vi "Instrument - Tool.vi"() -> ()   [LabVIEW 2019, in "Instrument Workspace Tool.lvlib"]
uses:
  Instrument Workspace Tool.lvlib
  NationalInstruments.VeriStand.SystemStorage
  Shared/Types/Response Wait Type.ctl
  Workspace Shared/Types/State Variables.ctl
  <vilib>/NI VeriStand/Display Template Support/DisplayTemplateSupport.llb/enum_Display Template Handler Minimal To Workspace.ctl
  <vilib>/NI VeriStand/Display Template Support/DisplayTemplateSupport.llb/enum_Display Template Handler Minimal To Widget Msg.ctl
  <vilib>/NI VeriStand/Execution/Workspace/WorkspaceAPI.ctl
  <vilib>/NI/STM/TCP/TCP Connection Info.ctl
  <vilib>/NI/STM/SubVIs/MetaDataElement.ctl
  Workspace Shared/Types/CD Saved State.ctl
  <vilib>/NI VeriStand/Execution/Workspace/SystemStateEventRef.ctl
  <vilib>/NI VeriStand/Execution/Workspace/Target State Info.ctl
  <vilib>/NI VeriStand/Execution/Workspace/Target State.ctl
  <vilib>/NI VeriStand/Execution/Workspace/SystemStateRegEventRef.ctl
  Shared/Types/Buffered RT Instrument Command.ctl
  <vilib>/NI VeriStand/Execution/Workspace/NI_VS Workspace ExecutionAPI.lvlib
  Host API/Instrument CD Host API.lvlib
  Shared/Instrument Addon Shared.lvlib
  <vilib>/NI/STM/NI STM.lvlib
  Workspace Shared/Instrument Workspace Shared.lvlib
  NationalInstruments.VeriStand.ClientAPI
panel:
  in  "Command":string
  in  "Response?":bool
  in  "Wait Type":T1
  in  "Wait Value":dbl=100.0 format="%#_p"
  out "Timed Out?":bool
  out "Error Report":errorcluster
  out "Response":string
  in  "Send":bool
  out "Device":string
  in  "NIVS.Gateway IP Address":string
  in  "NIVS.System Definition Root":refnum<k24>
  in  "NIVS.Workspace Event":refnum<event-registration>
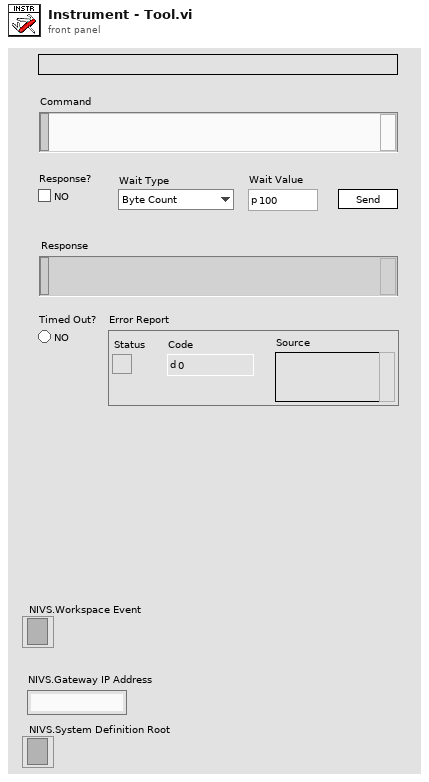
[diagram p1: front panel]
types:
  T1 = typedef "Instrument Addon Shared.lvlib/Response Wait Type.ctl" = enum16{"Byte Count", "Wait sec"}
  T2 = typedef "Instrument Workspace Shared.lvlib/State Variables.ctl" = cluster{"UI.Device":refnum<vi>, "NIVS.CachedDataRef":refnum<user-event>, "NIVS.LaunchRef":refnum<user-event>, "NIVS.SysDefRoot":refnum<k24>, "NIVS.Workspace":T3, "connection info":T4, "NIVS.CachedData":T6, "NIVS.SystemStateRefs":T7, "NIVS.UserEventRefs":cluster{"WorkspaceEvent":refnum<event-registration>, "SystemChangeEventRef":T8, "LaunchRef":refnum<event-registration>}, "Workspace.Connected?":bool, "NIVS.Workspace Event":refnum<event-registration>}
  T3 = typedef "NI_VS Workspace ExecutionAPI.lvlib/WorkspaceAPI.ctl" = refnum<k24>
  T4 = typedef "NI STM.lvlib/TCP Connection Info.ctl" = cluster{"connection ID":refnum<k5>, "meta data":T5[]}
  T5 = typedef "NI STM.lvlib/MetaDataElement.ctl" = string
  T6 = typedef "Instrument Workspace Shared.lvlib/CD Saved State.ctl" = cluster{"CD Path":string, "CD IP":string}
  T7 = typedef "NI_VS Workspace ExecutionAPI.lvlib/SystemStateEventRef.ctl" = cluster{"CustDatRef":refnum<user-event>, "EvtRef":refnum<k27>, "Target State User Event":refnum<user-event>}
  T8 = typedef "NI_VS Workspace ExecutionAPI.lvlib/SystemStateRegEventRef.ctl" = refnum<event-registration>
  T9 = typedef "enum_Display Template Handler Minimal To Workspace.ctl" = cluster{"Operation":enum16{"SetCustomData", "DeleteItem"}, "Data":variant}
  T10 = typedef "Instrument Addon Shared.lvlib/Buffered RT Instrument Command.ctl" = cluster{"Command":string, "Response Expected?":bool, "Wait Type":T1, "Wait Value":dbl}
  T11 = typedef "NI_VS Workspace ExecutionAPI.lvlib/SystemState.ctl" = u8
  T12 = enum8{"Enabled", "Disabled", "Disabled and Grayed Out"}
  T13 = cluster{"WorkspaceEvent":refnum<event-registration>, "SystemChangeEventRef":T8, "LaunchRef":refnum<event-registration>}
  T14 = typedef "enum_Display Template Handler Minimal To Widget Msg.ctl" = enum16{"Stop", "LaunchConfigDialog"}
  T15 = typedef "Instrument Addon Shared.lvlib/Buffered RT Instrument Request.ctl" = cluster{"Response":string, "Error":errorcluster}
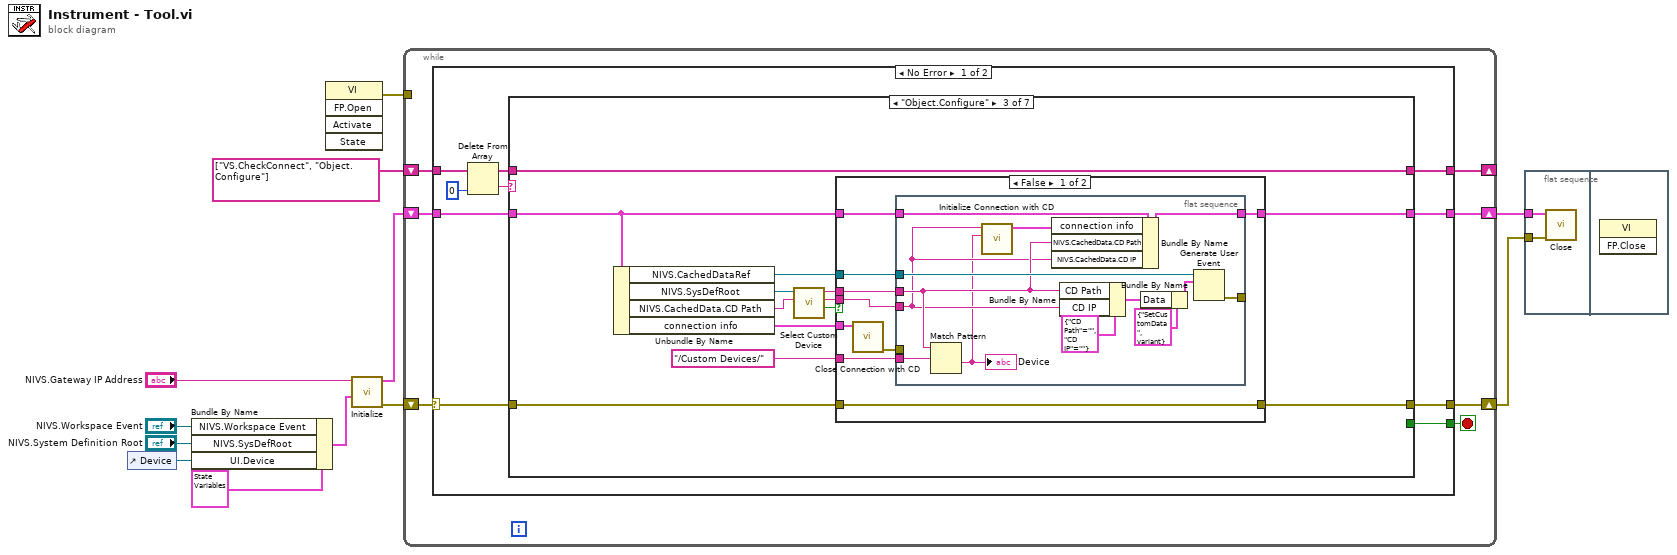
[diagram p0: block diagram]
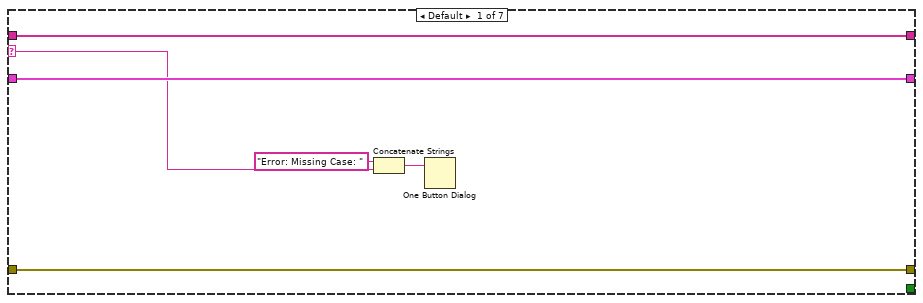
[diagram p2: hidden frame]
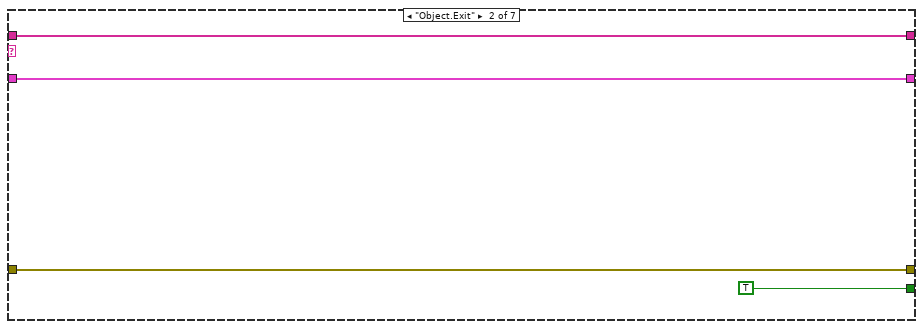
[diagram p3: hidden frame]
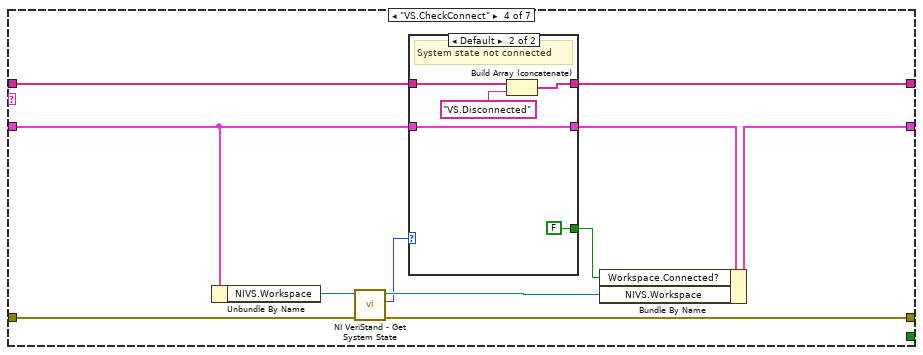
[diagram p5: hidden frame]
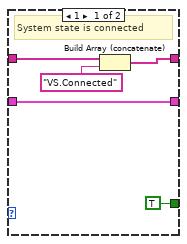
[diagram p6: hidden frame]
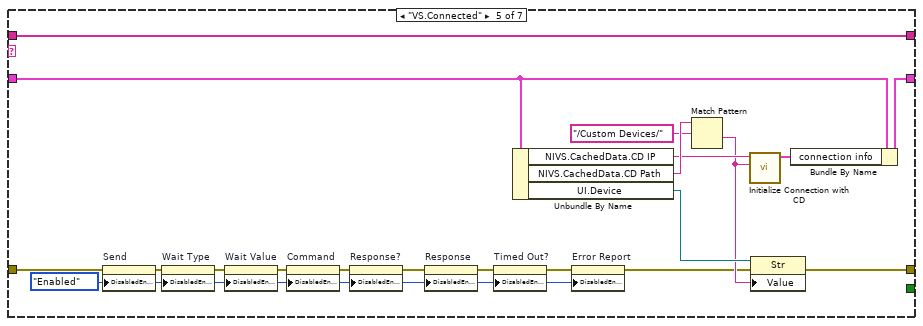
[diagram p7: hidden frame]
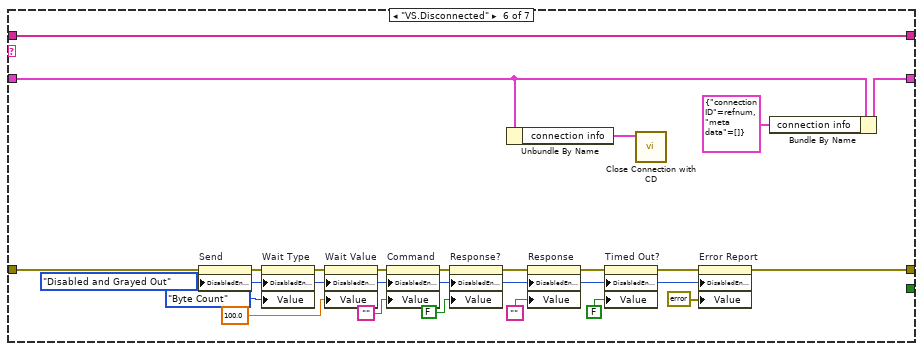
[diagram p8: hidden frame]
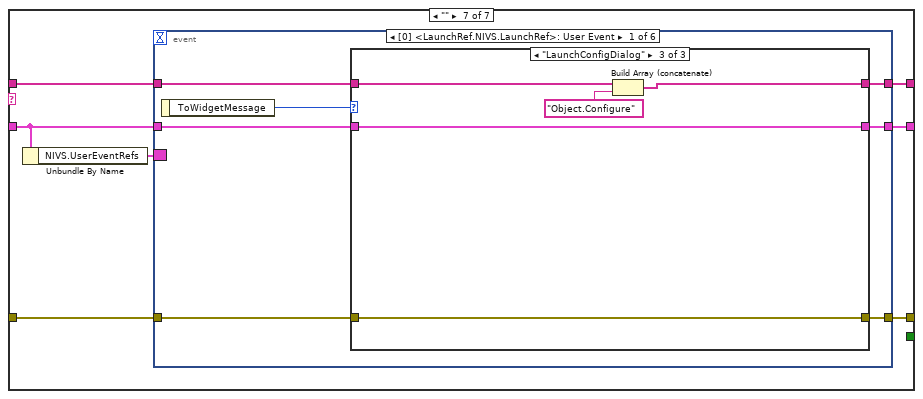
[diagram p9: hidden frame]
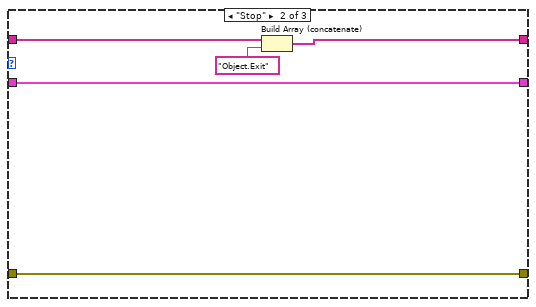
[diagram p11: hidden frame]
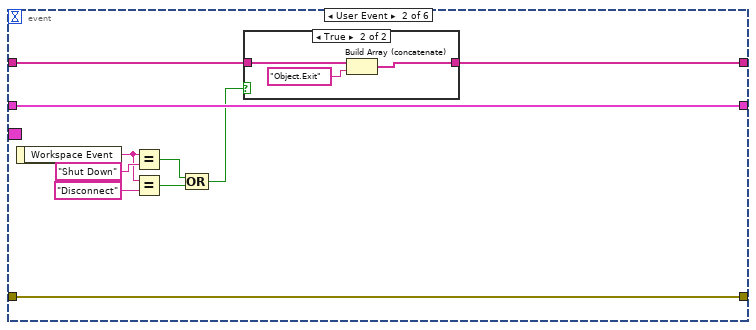
[diagram p12: hidden frame]
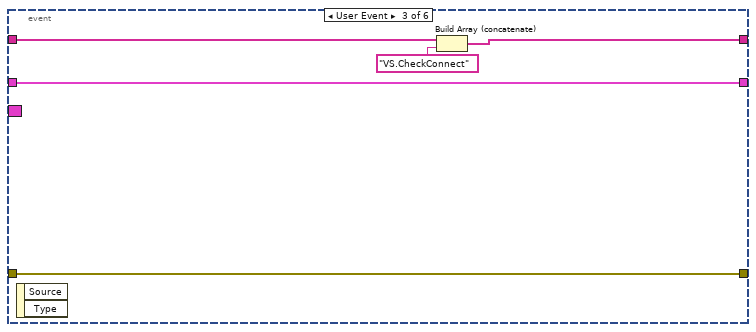
[diagram p14: hidden frame]
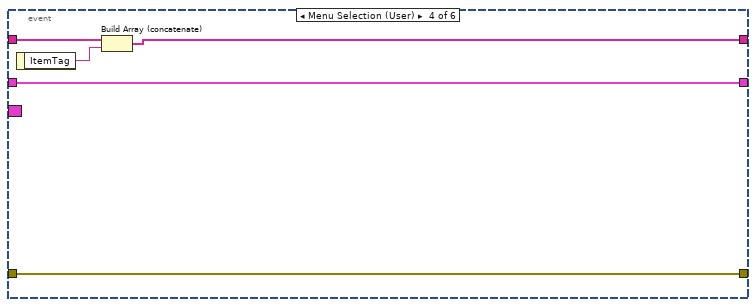
[diagram p15: hidden frame]
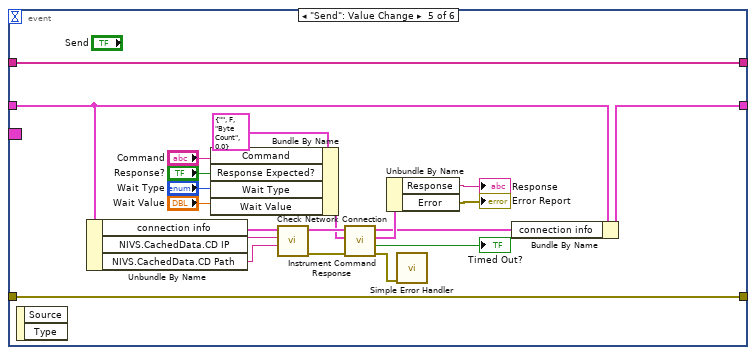
[diagram p16: hidden frame]
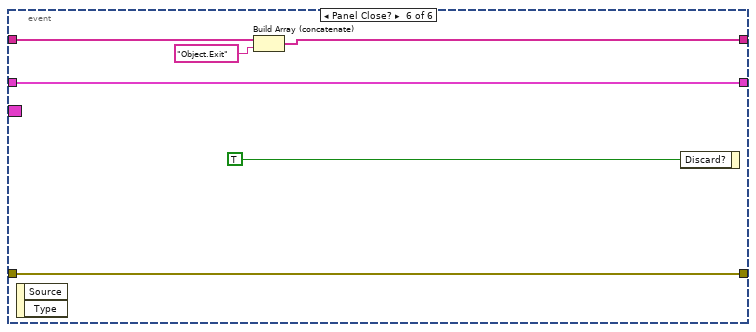
[diagram p17: hidden frame]
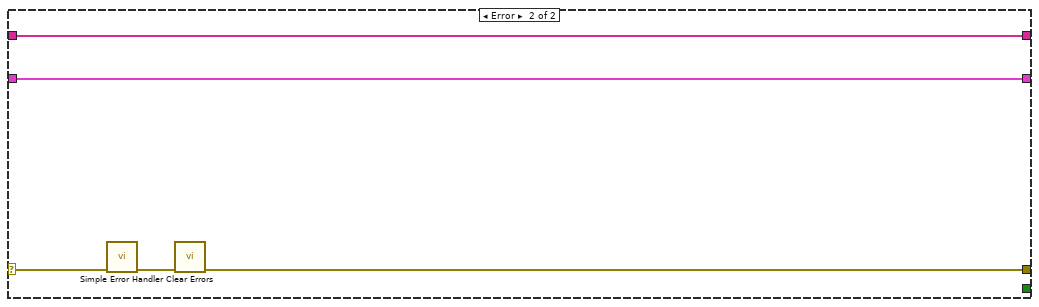
[diagram p18: hidden frame]
diagram:
  n1 = control-ref of="Device"() -> (w12:refnum<vi>)
  n2 = Bundle By Name(cluster=T2 {"UI.Device"=refnum, "NIVS.CachedDataRef"=refnum, "NIVS.LaunchRef"=refnum, "NIVS.SysDefRoot"=refnum, "NIVS.Workspace"=refnum, "connection info"={"connection ID"=refnum, "meta data"=[]}, "NIVS.CachedData"={"CD Path"="", "CD IP"=""}, "NIVS.SystemStateRefs"={"CustDatRef"=refnum, "EvtRef"=refnum, "Target State User Event"=refnum}, "NIVS.UserEventRefs"={"WorkspaceEvent"=refnum, "SystemChangeEventRef"=refnum, "LaunchRef"=refnum}, "Workspace.Connected?"=FALSE, "NIVS.Workspace Event"=refnum} ("State Variables in"), "NIVS.Workspace Event"="NIVS.Workspace Event", "NIVS.SysDefRoot"="NIVS.System Definition Root", "UI.Device"=w12) -> (w7:T2)
  n3 = invoke class="VI" method="FP.Open"() -> (error out=w9:errorcluster)  [unwired: 5 in, 4 out]
  n4 = call "Initialize.vi"("State Variables in"=w7, "NIVS.Gateway IP Address"="NIVS.Gateway IP Address") -> ("error out"=w6:errorcluster, "State Variables out"=w5:T2)  [unwired: 8 in]
  n5 = while {
    shift-right: [w18] -> w3
    shift-left: w6 -> [w15]
    shift-right: [w16] -> w4
    shift-left: w5 -> [w17]
    shift-right: [w13] -> _
    shift-left: string[] ["VS.CheckConnect", "Object.Configure"] -> [w14]
    tunnel: w9 -> [_]
    stop <- w19 stop-if-true
    n6 = case shown="No Error" w15 {
      selector: w15 -> [w25 w219]
      tunnel: [w29 _] -> w19
      tunnel: [w28 w218] -> w18
      tunnel: w17 -> [w27 w222]
      tunnel: [w26 w222] -> w16
      tunnel: w14 -> [w23 w221]
      tunnel: [w20 w221] -> w13
      frame No Error {
        n7 = Delete From Array(array=w23, index=0) -> (deleted portion=w22:string, array with subset deleted=w21:string[])  [unwired: 1 in]
        n8 = case shown="\"Object.Configure\"" w22 {
          selector: w22 -> [w32 _ _ _ _ _ _]
          tunnel: [_ TRUE _ _ _ _ _] -> w29
          tunnel: [w34 w38 w44 w80 w112 w122 w146] -> w28
          tunnel: w27 -> [w35 w39 w46 w82 w109 w136 w144]
          tunnel: [w35 w39 w43 w79 w108 w135 w143] -> w26
          tunnel: w25 -> [w34 w38 w48 w81 w117 w139 w142]
          tunnel: w21 -> [w33 w37 w47 w78 w116 w138 w140]
          tunnel: [w33 w37 w47 w77 w116 w138 w141] -> w20
          frame Default {
            n9 = Concatenate Strings("Error: Missing Case: " ("string"), w32) -> (w31:string)
            n10 = One Button Dialog(message=w31) -> ()  [unwired: 1 in, 1 out]
          }
          frame "Object.Exit" {
          }
          frame "Object.Configure" {
            n11 = Unbundle By Name(w46) -> ("NIVS.CachedDataRef"=w51:refnum<user-event>, "NIVS.SysDefRoot"=w52:refnum<k24>, "NIVS.CachedData.CD Path"=w49:string, "connection info"=w50:T4)
            n12 = call "Select Custom Device.vi"("CD Path"=w49, "NIVS.System Definition Root"=w52) -> ("Cancelled?"=w42:bool, "IP Address"=w41:string, "Custom Device Path Out"=w40:string)  [unwired: 7 in]
            n13 = case shown="False" w42 {
              tunnel: w51 -> [w61 _]
              tunnel: w41 -> [w58 _]
              tunnel: w40 -> [w59 _]
              tunnel: "/Custom Devices/" ("regular expression") -> [w60 _]
              tunnel: w50 -> [w57 _]
              tunnel: [w55 w76] -> w43
              tunnel: w46 -> [w54 w76]
              tunnel: [w53 w75] -> w44
              tunnel: w48 -> [w53 w75]
              frame False {
                n14 = call "Close Connection with CD.vi"("connection info"=w57) -> ("error out"=w56:errorcluster)  [unwired: 10 in]
                n15 = flat-sequence {
                  tunnel: w61 -> [w74]
                  tunnel: w60 -> [w71]
                  tunnel: w59 -> [w67]
                  tunnel: w58 -> [w66]
                  tunnel: w56 -> [_]
                  tunnel: [w69] -> w55
                  tunnel: w54 -> [w70]
                  tunnel: [w62] -> _
                  frame #0 {
                    n16 = Match Pattern(string=w67, regular expression=w71) -> (after substring=w63:string)  [unwired: 1 in, 3 out]
                    "Device" <- w63
                    n17 = call "Initialize Connection with CD.vi"("TCP Service"=w63, "IP Address"=w66) -> ("connection info out"=w65:T4)  [unwired: 8 in, 1 out]
                    n18 = Bundle By Name(cluster=w70, "connection info"=w65, "NIVS.CachedData.CD Path"=w67, "NIVS.CachedData.CD IP"=w66) -> (w69:T2)
                    n19 = Bundle By Name(cluster=T6 {"CD Path"="", "CD IP"=""}, "CD Path"=w67, "CD IP"=w66) -> (w64:T6)
                    n20 = Bundle By Name(cluster=T9 {"Operation"=enum."SetCustomData", "Data"=variant} ("event data"), "Data"=w64) -> (w72:T9)
                    n21 = Generate User Event(user event=w74, event data cluster=w72) -> (error out=w62:errorcluster)  [unwired: 2 in, 1 out]
                  }
                }
              }
              frame True {
              }
            }
          }
          frame "VS.CheckConnect" {
            n22 = Unbundle By Name(w82) -> ("NIVS.Workspace"=w86:T3)
            n23 = call <vilib>:"NI VeriStand - Get System State.vi"("error in (no error)"=w81, "WorkspaceManager in"=w86) -> ("error out"=w80:errorcluster, "System State"=w83:T11, "WorkspaceManager  out"=w87:T3)  [unwired: 5 in, 2 out]
            n24 = case shown="Default" w83 {
              tunnel: [w92 w97] -> w77
              tunnel: [w90 w95] -> w84
              tunnel: w82 -> [w90 w95]
              tunnel: [TRUE FALSE] -> w85
              tunnel: w78 -> [w88 w93]
              frame 1 {
                # "System state is connected"
                n25 = Build Array (concatenate)(w88, "VS.Connected") -> (w92:string[])
              }
              frame Default {
                # "System state not connected"
                n26 = Build Array (concatenate)(w93, "VS.Disconnected") -> (w97:string[])
              }
            }
            n27 = Bundle By Name(cluster=w84, "Workspace.Connected?"=w85, "NIVS.Workspace"=w87) -> (w79:T2)
          }
          frame "VS.Connected" {
            w98 = T12."Enabled" ("Disabled")
            n28 = property on="Send" class="Bool"(error in=w117, "DisabledEnum"=w98) -> (error out=w104:errorcluster)  [unwired: 1 in, 1 out]
            n29 = property on="Wait Type" class="Enum (strict)"(error in=w104, "DisabledEnum"=w98) -> (error out=w107:errorcluster)  [unwired: 1 in, 1 out]
            n30 = property on="Wait Value" class="DigNum (strict)"(error in=w107, "DisabledEnum"=w98) -> (error out=w106:errorcluster)  [unwired: 1 in, 1 out]
            n31 = property on="Command" class="Str"(error in=w106, "DisabledEnum"=w98) -> (error out=w105:errorcluster)  [unwired: 1 in, 1 out]
            n32 = property on="Response?" class="Bool (strict)"(error in=w105, "DisabledEnum"=w98) -> (error out=w100:errorcluster)  [unwired: 1 in, 1 out]
            n33 = property on="Response" class="Str"(error in=w100, "DisabledEnum"=w98) -> (error out=w101:errorcluster)  [unwired: 1 in, 1 out]
            n34 = property on="Timed Out?" class="Bool (strict)"(error in=w101, "DisabledEnum"=w98) -> (error out=w102:errorcluster)  [unwired: 1 in, 1 out]
            n35 = Unbundle By Name(w109) -> ("NIVS.CachedData.CD IP"=w114:string, "NIVS.CachedData.CD Path"=w115:string, "UI.Device"=w111:refnum<vi>)
            n36 = property on="Error Report" class="Clust (strict)"(error in=w102, "DisabledEnum"=w98) -> (error out=w99:errorcluster)  [unwired: 1 in, 1 out]
            n37 = Match Pattern(string=w115, regular expression="/Custom Devices/") -> (after substring=w103:string)  [unwired: 1 in, 3 out]
            n38 = call "Initialize Connection with CD.vi"("TCP Service"=w103, "IP Address"=w114) -> ("connection info out"=w110:T4)  [unwired: 8 in, 1 out]
            n39 = property class="Str"(reference=w111, error in=w99, "Value"=w103) -> (error out=w112:errorcluster)  [unwired: 1 out]
            n40 = Bundle By Name(cluster=w109, "connection info"=w110) -> (w108:T2)
          }
          frame "VS.Disconnected" {
            w121 = T12."Disabled and Grayed Out" ("Disabled")
            n41 = property on="Send" class="Bool"(error in=w139, "DisabledEnum"=w121) -> (error out=w131:errorcluster)  [unwired: 1 in, 1 out]
            n42 = property on="Wait Type" class="Enum (strict)"(error in=w131, "DisabledEnum"=w121, "Value"=Response_Wait_Type."Byte Count" ("Wait Type")) -> (error out=w134:errorcluster)  [unwired: 1 in, 1 out]
            n43 = property on="Wait Value" class="DigNum (strict)"(error in=w134, "DisabledEnum"=w121, "Value"=100.0 ("Wait Value")) -> (error out=w133:errorcluster)  [unwired: 1 in, 1 out]
            n44 = property on="Command" class="Str"(error in=w133, "DisabledEnum"=w121, "Value"="") -> (error out=w132:errorcluster)  [unwired: 1 in, 1 out]
            n45 = property on="Response?" class="Bool (strict)"(error in=w132, "DisabledEnum"=w121, "Value"=FALSE ("Response?")) -> (error out=w123:errorcluster)  [unwired: 1 in, 1 out]
            n46 = Unbundle By Name(w136) -> ("connection info"=w137:T4)
            n47 = property on="Response" class="Str"(error in=w123, "DisabledEnum"=w121, "Value"="") -> (error out=w124:errorcluster)  [unwired: 1 in, 1 out]
            n48 = property on="Timed Out?" class="Bool (strict)"(error in=w124, "DisabledEnum"=w121, "Value"=FALSE ("Response?")) -> (error out=w125:errorcluster)  [unwired: 1 in, 1 out]
            n49 = call "Close Connection with CD.vi"("connection info"=w137) -> ()  [unwired: 10 in, 1 out]
            n50 = property on="Error Report" class="Clust (strict)"(error in=w125, "DisabledEnum"=w121, "Value"=errorcluster {"Status"=FALSE, "Code"=0, "Source"=""} ("Error Report")) -> (error out=w122:errorcluster)  [unwired: 1 in, 1 out]
            n51 = Bundle By Name(cluster=w136, "connection info"=T4 {"connection ID"=refnum, "meta data"=[]}) -> (w135:T2)
          }
          frame "" {
            n52 = Unbundle By Name(w144) -> ("NIVS.UserEventRefs"=w145:T13)
            n53 = event shown="[0] <LaunchRef.NIVS.LaunchRef>: User Event" {
              selector: w145 -> [_ _ _ _ _ _]
              dyn-events: _ -> [_ _ _ _ _ _]
              timeout: _ -> [_ _ _ _ _ _]
              tunnel: [w152 w172 w182 w187 w193 w217] -> w143
              tunnel: w142 -> [w149 w167 w181 w186 w192 w216]
              tunnel: [w150 w167 w181 w186 w192 w216] -> w146
              tunnel: w144 -> [w151 w172 w182 w187 w194 w217]
              tunnel: [w148 w170 w183 w188 w191 w214] -> w141
              tunnel: w140 -> [w147 w169 w184 w190 w191 w213]
              event User Event {
                n54 = event-data() -> ("ToWidgetMessage"=w153:T14)  [unwired: 1 out]
                n55 = case shown="\"LaunchConfigDialog\"" w153 {
                  tunnel: [w156 w161 w166] -> w152
                  tunnel: w151 -> [w156 w161 w166]
                  tunnel: [w155 w160 w165] -> w150
                  tunnel: w149 -> [w155 w160 w165]
                  tunnel: [w154 w158 w164] -> w148
                  tunnel: w147 -> [w154 w157 w163]
                  frame Default {
                  }
                  frame "Stop" {
                    n56 = Build Array (concatenate)(w157, "Object.Exit") -> (w158:string[])
                  }
                  frame "LaunchConfigDialog" {
                    n57 = Build Array (concatenate)(w163, "Object.Configure") -> (w164:string[])
                  }
                }
              }
              event User Event {
                n58 = event-data() -> ("Workspace Event"=w168:string)  [unwired: 1 out]
                n59 = Equal?(x=w168, y="Shut Down") -> (x = y?=w173:bool)
                n60 = Equal?(x=w168, y="Disconnect") -> (x = y?=w174:bool)
                n61 = Compound Arithmetic op=OR(w173, w174) -> (w171:bool)
                n62 = case shown="True" w171 {
                  tunnel: [w177 w179] -> w170
                  tunnel: w169 -> [w177 w178]
                  frame False {
                  }
                  frame True {
                    n63 = Build Array (concatenate)(w178, "Object.Exit") -> (w179:string[])
                  }
                }
              }
              event User Event {
                n64 = event-data() -> ()  [unwired: 3 out]
                n65 = Build Array (concatenate)(w184, "VS.CheckConnect") -> (w183:string[])
              }
              event Menu Selection (User) {
                n66 = event-data() -> ("ItemTag"=w189:string)  [unwired: 1 out]
                n67 = Build Array (concatenate)(w190, w189) -> (w188:string[])
              }
              event "Send": Value Change {
                n68 = event-data() -> ()  [unwired: 3 out]
                n69 = Unbundle By Name(w194) -> ("connection info"=w196:T4, "NIVS.CachedData.CD IP"=w211:string, "NIVS.CachedData.CD Path"=w210:string)
                n70 = Bundle By Name(cluster=T10 {"Command"="", "Response Expected?"=FALSE, "Wait Type"=enum."Byte Count", "Wait Value"=0.0} ("Command Parameters"), "Command"="Command", "Response Expected?"="Response?", "Wait Type"="Wait Type", "Wait Value"="Wait Value") -> (w203:T10)
                n71 = call "Check Network Connection.vi"("CD Path"=w210, "IP Address"=w211, "connection info"=w196) -> ("error out"=w208:errorcluster, "connection info"=w209:T4)  [unwired: 7 in]
                n72 = call "Instrument Command Response.vi"("error in (no error)"=w208, "Command Parameters"=w203, "connection info"=w209) -> ("error out"=w198:errorcluster, "Timed Out?"=→"Timed Out?":bool, "Response"=w201:T15, "connection info"=w195:T4)  [unwired: 5 in]
                n73 = Unbundle By Name(w201) -> ("Response"=→"Response":string, "Error"=→"Error Report":errorcluster)
                n74 = call <vilib>:"Simple Error Handler.vi"("error in (no error)"=w198) -> ()  [unwired: 4 in, 5 out]
                n75 = Bundle By Name(cluster=w194, "connection info"=w195) -> (w193:T2)
              }
              event Panel Close? {
                n76 = event-data() -> ()  [unwired: 3 out]
                n77 = Build Array (concatenate)(w213, "Object.Exit") -> (w214:string[])
                n78 = event-data("Discard?"=TRUE) -> ()  [unwired: 1 in, 1 out]
              }
            }
          }
        }
      }
      frame Error {
        n79 = call <vilib>:"Simple Error Handler.vi"("error in (no error)"=w219) -> ("error out"=w220:errorcluster)  [unwired: 4 in, 4 out]
        n80 = call <vilib>:"Clear Errors.vi"("error in (no error)"=w220) -> ("error out"=w218:errorcluster)  [unwired: 5 in, 1 out]
      }
    }
  }
  n81 = flat-sequence {
    tunnel: w3 -> [w224]
    tunnel: w4 -> [w223]
    frame #0 {
      n82 = call "Close.vi"("error in (no error)"=w224, "State Variables in"=w223) -> ()  [unwired: 10 in]
    }
    frame #1 {
      n83 = invoke class="VI" method="FP.Close"() -> ()  [unwired: 3 in, 3 out]
    }
  }
